vi "Replace Command with Cached Command.vi"(9 "Cached Commands":T1, 10 "Name":string, 11 "VI in":refnum<vi>) -> (3 "VI out":refnum<vi>)   [LabVIEW 2025]
uses:
  Types/Command Editor Info.ctl
  Types/Single Cmd Info.ctl
  <vilib>/picture/picture.llb/imagedata.ctl
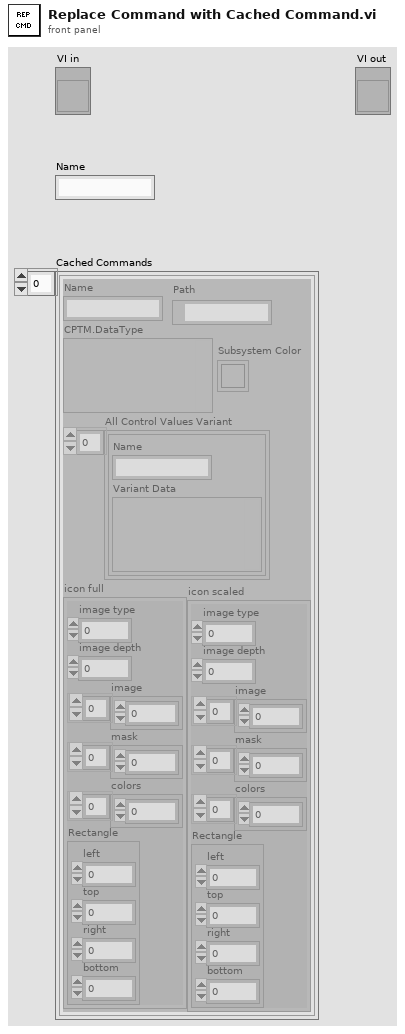
[diagram p1: front panel]
types:
  T1 = typedef "Command Editor Info.ctl" = T2[]
  T2 = typedef "Single Cmd Info.ctl" = cluster{"Name":string, "CPTM.DataType":variant, "All Control Values Variant":cluster{"Name":string, "Variant Data":variant}[], "icon full":T3, "icon scaled":T3, "Path":path, "Subsystem Color":u32}
  T3 = typedef "imagedata.ctl" = cluster{"image type":i32, "image depth":i32, "image":u8[], "mask":u8[], "colors":u32[], "Rectangle":cluster{"left":i16, "top":i16, "right":i16, "bottom":i16}}
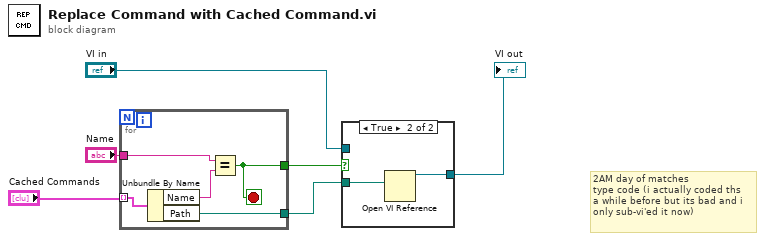
[diagram p0: block diagram]
diagram:
  # "2AM day of matches\ntype code (i actually coded ths\na while before but its bad and i\nonly sub-vi'ed it now)"
  n1 = for {
    tunnel: "Cached Commands" -> [w11] mode=indexing
    tunnel: "Name" -> [w9]
    tunnel: [w8] -> w3
    tunnel: [w7] -> w4
    stop <- w8 stop-if-true
    n2 = Unbundle By Name(w11) -> ("Name"=w10:string, "Path"=w7:path)
    n3 = Equal?(x=w9, y=w10) -> (x = y?=w8:bool)
  }
  n4 = case shown="True" w3 {
    tunnel: w4 -> [_ w14]
    tunnel: [w12 w13] -> w5
    tunnel: "VI in" -> [w12 _]
    frame False {
    }
    frame True {
      n5 = Open VI Reference(vi path=w14) -> (vi reference=w13:refnum<vi>)  [unwired: 5 in, 1 out]
    }
  }
  "VI out" <- w5
